vi "DAQ.Create.vi"(8 "error in (no error)":errorcluster, 11 "Instrument.DAQ in":refnum<class "Instrument.DAQ.lvclass">) -> (0 "error out":errorcluster, 3 "Instrument.DAQ out":refnum<class "Instrument.DAQ.lvclass">)   [LabVIEW 2019, in "Instrument.Lockin.lvlib" / "Instrument.DAQ.lvclass"]
uses:
  Instrument.DAQ.lvclass
  Instrument.DAQ.lvclass/Instrument.DAQ.ctl
  DAQmx/DAQmx.lvclass
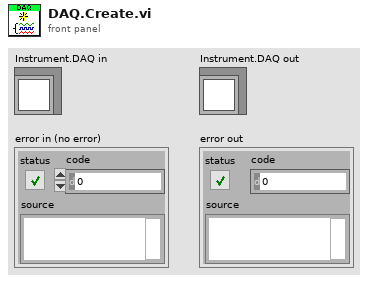
[diagram p1: front panel]
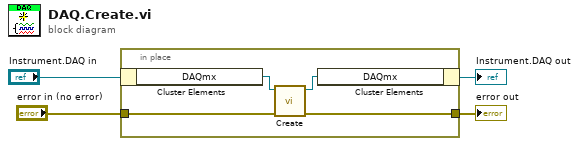
[diagram p0: block diagram]
diagram:
  n1 = in-place {
    in-place-border: [w8] -> w4
    in-place-border: "error in (no error)" -> [w7]
    n2 = in-place-cluster #1("Instrument.DAQ in") -> ("DAQmx"=w6:refnum<class "DAQmx.lvclass">)
    n3 = call "Create.vi"("error in"=w7, "DAQmx in"=w6) -> ("error out"=w8:errorcluster, "DAQmx out"=w5:refnum<class "DAQmx.lvclass">)  [unwired: 8 in]
    n4 = in-place-cluster #1("DAQmx"=w5) -> (→"Instrument.DAQ out":refnum<class "Instrument.DAQ.lvclass">)
  }
  "error out" <- w4
